vi "DI Notifier.vi"(11 "Action":enum16{"Get", "Set"}(ring)) -> (3 "Trigger?":bool)   [LabVIEW 2021]
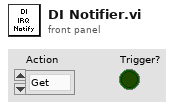
[diagram p1: front panel]
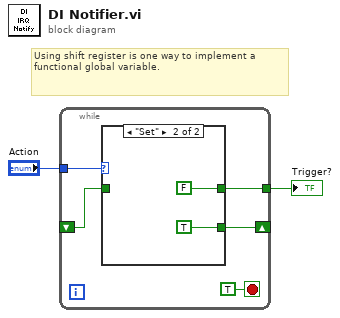
[diagram p0: block diagram]
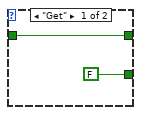
[diagram p2: hidden frame]
diagram:
  # "Using shift register is one way to implement a functional global variable."
  n1 = while {
    tunnel: [w7] -> w2
    tunnel: "Action" -> [w6]
    shift-right: [w4] -> _
    shift-left: _ -> [w5]
    stop <- TRUE stop-if-true
    n2 = case shown="\"Set\"" w6 {
      tunnel: [w9 FALSE ("Boolean")] -> w7
      tunnel: [FALSE TRUE] -> w4
      tunnel: w5 -> [w9 _]
      frame "Get" {
      }
      frame "Set" {
      }
    }
  }
  "Trigger?" <- w2
